vi "Round Settings.vi"(7 "DG_Number":i32, 8 "error in (no error)":errorcluster, 11 "Settings":T1={"Channel A"={"Delay (µs)"=0.013000000000000001, "Pulse Width (µs)"=0.019, "Output Modulo"=300, "Output Offset"=0, "Go Signal"=16, "Polarity"=TRUE, "Terminate"=FALSE}, "Channel B"={"Delay (µs)"=0.032, "Pulse Width (µs)"=0.019, "Output Modulo"=300, "Output Offset"=0, "Go Signal"=16, "Polarity"=TRUE, "Terminate"=FALSE}, "Channel C"={"Delay (µs)"=0.0, "Pulse Width (µs)"=0.01, "Output Modulo"=300, "Output Offset"=0, "Go Signal"=16, "Polarity"=TRUE, "Terminate"=FALSE}, "Channel D"={"Delay (µs)"=0.01, "Pulse Width (µs)"=0.01, "Output Modulo"=300, "Output Offset"=0, "Go Signal"=16, "Polarity"=TRUE, "Terminate"=FALSE}, "Channel E"={"Delay (µs)"=0.039999999999999994, "Pulse Width (µs)"=0.01, "Output Modulo"=300, "Output Offset"=1, "Go Signal"=16, "Polarity"=TRUE, "Terminate"=FALSE, "Disconnect"=FALSE, "Onto MsBus"=FALSE, "Input Positive"=TRUE}, "Channel F"={"Delay (µs)"=0.04999999999999999, "Pulse Width (µs)"=0.01, "Output Modulo"=300, "Output Offset"=1, "Go Signal"=16, "Polarity"=TRUE, "Terminate"=FALSE, "Disconnect"=FALSE, "Onto MsBus"=FALSE, "Input Positive"=TRUE}, "Clock Enable"=TRUE, "Ocillator Divider"=2, "Trigger Divider"=1, "Trigger Multiplier"=4, "Clock Source"=3, "Trigger Terminate"=TRUE, "Gate Terminate"=TRUE, "Trigger Level"=0.2, "Gate Level"=0.0, "Gate Delay (µs)"=-1.0, "MS Bus"=1, "Internal Clock (µs)"=0.0083333, "Stop Trigger"=1, "Gate Divider"=0, "Force Trigger (µs)"=-1.0, "Step Back Time (µs)"=-1.0, "Burst Counter"=1, "Positive Gate"=TRUE, "Trigger Source"=TRUE, "Gate Type"=TRUE, "Synchronize Gate"=FALSE, "Trigger Slope"=TRUE, "Stop on Preset"=FALSE, "Reset When Done"=TRUE, "Trigger Enable"=TRUE, "Gate AB"=0, "Gate CD"=0, "Gate EF"=0} {"Gate EF" items=["Normal"=0, "EF_OR"=1048576, "EF_AND"=2097152, "EF_XOR"=3145728]; "Gate CD" items=["Normal"=0, "CD_OR"=262144, "CD_AND"=524288, "CD_XOR"=786432]; "Gate AB" items=["Normal"=0, "AB_OR"=65536, "AB_AND"=131072, "AB_XOR"=196608]; "Step Back Time (µs)" min=-1.0 format="%.6f"; "Force Trigger (µs)" min=-1.0 format="%.6f"; "Gate Delay (µs)" min=-1.0 format="%.6f"; "Internal Clock (µs)" min=0.0 format="%.6f"; "MS Bus" format="%04x" items=["Local Primary"=1, "Local Secondary"=2, "Local Force"=4, "Resynchronize"=8, "Master Primary"=16, "Master Secondary"=32, "Master Force"=64, "System Clock"=128, "Delay Clock"=256, "Inhibit Local"=512, "Start Local"=1024, "Start Bus"=2048, "Step Back Local"=4096, "Step Back Bus"=8192, "Enable From E"=65536, "Enable From F"=131072, "Enable From Bus"=262144]; "Gate Level" min=-2.5 max=2.5 format="%.3g"; "Trigger Level" min=-2.5 max=2.5 format="%.3f"; "Clock Source" items=["Internal Oscillator"=1, "External Trigger"=2, "Trigger & Oscillator"=3, "Master Slave Bus"=4]; "Trigger Multiplier" min=1; "Trigger Divider" min=1; "Ocillator Divider" min=1; "Channel F"."Go Signal" format="%04x" items=["Loc Prim"=1, "Loc Sec"=2, "Loc Force"=4, "Resynch"=8, "Mas Prim"=16, "Mas Sec"=32, "Mas Force"=64, "Sys Clock"=128, "Delay Clock"=256, "Inhibit Local"=512, "Start Local"=1024, "Start Bus"=2048, "Step Back Loc"=4096, "Step Back Bus"=8192, "From E"=65536, "From F"=131072, "From Bus"=262144]; "Channel F"."Pulse Width (µs)" min=0.0 max=8947840.0 format="%.6f"; "Channel F"."Delay (µs)" min=0.0 format="%.6f"; "Channel E"."Go Signal" format="%04x" items=["Loc Prim"=1, "Loc Sec"=2, "Loc Force"=4, "Resynch"=8, "Mas Prim"=16, "Mas Sec"=32, "Mas Force"=64, "Sys Clock"=128, "Delay Clock"=256, "Inhibit Local"=512, "Start Local"=1024, "Start Bus"=2048, "Step Back Loc"=4096, "Step Back Bus"=8192, "From E"=65536, "From F"=131072, "From Bus"=262144]; "Channel E"."Pulse Width (µs)" min=0.0 max=8947840.0 format="%.6f"; "Channel E"."Delay (µs)" min=0.0 format="%.6f"; "Channel D"."Go Signal" format="%04x" items=["Loc Prim"=1, "Loc Sec"=2, "Loc Force"=4, "Resynch"=8, "Mas Prim"=16, "Mas Sec"=32, "Mas Force"=64, "Sys Clock"=128, "Delay Clock"=256, "Inhibit Local"=512, "Start Local"=1024, "Start Bus"=2048, "Step Back Loc"=4096, "Step Back Bus"=8192, "From E"=65536, "From F"=131072, "From Bus"=262144]; "Channel D"."Pulse Width (µs)" min=0.0 max=8947840.0 format="%.6f"; "Channel D"."Delay (µs)" min=0.0 format="%.6f"; "Channel C"."Go Signal" format="%04x" items=["Loc Prim"=1, "Loc Sec"=2, "Loc Force"=4, "Resynch"=8, "Mas Prim"=16, "Mas Sec"=32, "Mas Force"=64, "Sys Clock"=128, "Delay Clock"=256, "Inhibit Local"=512, "Start Local"=1024, "Start Bus"=2048, "Step Back Loc"=4096, "Step Back Bus"=8192, "From E"=65536, "From F"=131072, "From Bus"=262144]; "Channel C"."Pulse Width (µs)" min=0.0 max=8947840.0 format="%.6f"; "Channel C"."Delay (µs)" min=0.0 format="%.6f"; "Channel B"."Go Signal" format="%04x" items=["Loc Prim"=1, "Loc Sec"=2, "Loc Force"=4, "Resynch"=8, "Mas Prim"=16, "Mas Sec"=32, "Mas Force"=64, "Sys Clock"=128, "Delay Clock"=256, "Inhibit Local"=512, "Start Local"=1024, "Start Bus"=2048, "Step Back Loc"=4096, "Step Back Bus"=8192, "From E"=65536, "From F"=131072, "From Bus"=262144]; "Channel B"."Pulse Width (µs)" min=0.0 max=8947840.0 format="%.6f"; "Channel B"."Delay (µs)" min=0.0 format="%.6f"; "Channel A"."Go Signal" format="%04x" items=["Loc Prim"=1, "Loc Sec"=2, "Loc Force"=4, "Resynch"=8, "Mas Prim"=16, "Mas Sec"=32, "Mas Force"=64, "Sys Clock"=128, "Delay Clock"=256, "Inhibit Local"=512, "Start Local"=1024, "Start Bus"=2048, "Step Back Loc"=4096, "Step Back Bus"=8192, "From E"=65536, "From F"=131072, "From Bus"=262144]; "Channel A"."Pulse Width (µs)" min=0.0 max=8947840.0 format="%.6f"; "Channel A"."Delay (µs)" min=0.0 format="%.6f"}) -> (0 "error out":errorcluster, 3 "Settings":T1={"Channel A"={"Delay (µs)"=0.013000000000000001, "Pulse Width (µs)"=0.019, "Output Modulo"=300, "Output Offset"=0, "Go Signal"=16, "Polarity"=TRUE, "Terminate"=FALSE}, "Channel B"={"Delay (µs)"=0.032, "Pulse Width (µs)"=0.019, "Output Modulo"=300, "Output Offset"=0, "Go Signal"=16, "Polarity"=TRUE, "Terminate"=FALSE}, "Channel C"={"Delay (µs)"=0.0, "Pulse Width (µs)"=0.01, "Output Modulo"=300, "Output Offset"=0, "Go Signal"=16, "Polarity"=TRUE, "Terminate"=FALSE}, "Channel D"={"Delay (µs)"=0.01, "Pulse Width (µs)"=0.01, "Output Modulo"=300, "Output Offset"=0, "Go Signal"=16, "Polarity"=TRUE, "Terminate"=FALSE}, "Channel E"={"Delay (µs)"=0.039999999999999994, "Pulse Width (µs)"=0.01, "Output Modulo"=300, "Output Offset"=1, "Go Signal"=16, "Polarity"=TRUE, "Terminate"=FALSE, "Disconnect"=FALSE, "Onto MsBus"=FALSE, "Input Positive"=TRUE}, "Channel F"={"Delay (µs)"=0.04999999999999999, "Pulse Width (µs)"=0.01, "Output Modulo"=300, "Output Offset"=1, "Go Signal"=16, "Polarity"=TRUE, "Terminate"=FALSE, "Disconnect"=FALSE, "Onto MsBus"=FALSE, "Input Positive"=TRUE}, "Clock Enable"=TRUE, "Ocillator Divider"=2, "Trigger Divider"=1, "Trigger Multiplier"=4, "Clock Source"=3, "Trigger Terminate"=TRUE, "Gate Terminate"=TRUE, "Trigger Level"=0.2, "Gate Level"=0.0, "Gate Delay (µs)"=-1.0, "MS Bus"=1, "Internal Clock (µs)"=0.0083333, "Stop Trigger"=1, "Gate Divider"=0, "Force Trigger (µs)"=-1.0, "Step Back Time (µs)"=-1.0, "Burst Counter"=1, "Positive Gate"=TRUE, "Trigger Source"=TRUE, "Gate Type"=TRUE, "Synchronize Gate"=FALSE, "Trigger Slope"=TRUE, "Stop on Preset"=FALSE, "Reset When Done"=TRUE, "Trigger Enable"=TRUE, "Gate AB"=0, "Gate CD"=0, "Gate EF"=0} {"Gate EF" items=["Normal"=0, "EF_OR"=1048576, "EF_AND"=2097152, "EF_XOR"=3145728]; "Gate CD" items=["Normal"=0, "CD_OR"=262144, "CD_AND"=524288, "CD_XOR"=786432]; "Gate AB" items=["Normal"=0, "AB_OR"=65536, "AB_AND"=131072, "AB_XOR"=196608]; "Step Back Time (µs)" min=-1.0 format="%.6f"; "Force Trigger (µs)" min=-1.0 format="%.6f"; "Gate Delay (µs)" min=-1.0 format="%.6f"; "Internal Clock (µs)" min=0.0 format="%.6f"; "MS Bus" format="%04x" items=["Local Primary"=1, "Local Secondary"=2, "Local Force"=4, "Resynchronize"=8, "Master Primary"=16, "Master Secondary"=32, "Master Force"=64, "System Clock"=128, "Delay Clock"=256, "Inhibit Local"=512, "Start Local"=1024, "Start Bus"=2048, "Step Back Local"=4096, "Step Back Bus"=8192, "Enable From E"=65536, "Enable From F"=131072, "Enable From Bus"=262144]; "Gate Level" min=-2.5 max=2.5 format="%.3g"; "Trigger Level" min=-2.5 max=2.5 format="%.3f"; "Clock Source" items=["Internal Oscillator"=1, "External Trigger"=2, "Trigger & Oscillator"=3, "Master Slave Bus"=4]; "Trigger Multiplier" min=1; "Trigger Divider" min=1; "Ocillator Divider" min=1; "Channel F"."Go Signal" format="%04x" items=["Loc Prim"=1, "Loc Sec"=2, "Loc Force"=4, "Resynch"=8, "Mas Prim"=16, "Mas Sec"=32, "Mas Force"=64, "Sys Clock"=128, "Delay Clock"=256, "Inhibit Local"=512, "Start Local"=1024, "Start Bus"=2048, "Step Back Loc"=4096, "Step Back Bus"=8192, "From E"=65536, "From F"=131072, "From Bus"=262144]; "Channel F"."Pulse Width (µs)" min=0.0 max=8947840.0 format="%.6f"; "Channel F"."Delay (µs)" min=0.0 format="%.6f"; "Channel E"."Go Signal" format="%04x" items=["Loc Prim"=1, "Loc Sec"=2, "Loc Force"=4, "Resynch"=8, "Mas Prim"=16, "Mas Sec"=32, "Mas Force"=64, "Sys Clock"=128, "Delay Clock"=256, "Inhibit Local"=512, "Start Local"=1024, "Start Bus"=2048, "Step Back Loc"=4096, "Step Back Bus"=8192, "From E"=65536, "From F"=131072, "From Bus"=262144]; "Channel E"."Pulse Width (µs)" min=0.0 max=8947840.0 format="%.6f"; "Channel E"."Delay (µs)" min=0.0 format="%.6f"; "Channel D"."Go Signal" format="%04x" items=["Loc Prim"=1, "Loc Sec"=2, "Loc Force"=4, "Resynch"=8, "Mas Prim"=16, "Mas Sec"=32, "Mas Force"=64, "Sys Clock"=128, "Delay Clock"=256, "Inhibit Local"=512, "Start Local"=1024, "Start Bus"=2048, "Step Back Loc"=4096, "Step Back Bus"=8192, "From E"=65536, "From F"=131072, "From Bus"=262144]; "Channel D"."Pulse Width (µs)" min=0.0 max=8947840.0 format="%.6f"; "Channel D"."Delay (µs)" min=0.0 format="%.6f"; "Channel C"."Go Signal" format="%04x" items=["Loc Prim"=1, "Loc Sec"=2, "Loc Force"=4, "Resynch"=8, "Mas Prim"=16, "Mas Sec"=32, "Mas Force"=64, "Sys Clock"=128, "Delay Clock"=256, "Inhibit Local"=512, "Start Local"=1024, "Start Bus"=2048, "Step Back Loc"=4096, "Step Back Bus"=8192, "From E"=65536, "From F"=131072, "From Bus"=262144]; "Channel C"."Pulse Width (µs)" min=0.0 max=8947840.0 format="%.6f"; "Channel C"."Delay (µs)" min=0.0 format="%.6f"; "Channel B"."Go Signal" format="%04x" items=["Loc Prim"=1, "Loc Sec"=2, "Loc Force"=4, "Resynch"=8, "Mas Prim"=16, "Mas Sec"=32, "Mas Force"=64, "Sys Clock"=128, "Delay Clock"=256, "Inhibit Local"=512, "Start Local"=1024, "Start Bus"=2048, "Step Back Loc"=4096, "Step Back Bus"=8192, "From E"=65536, "From F"=131072, "From Bus"=262144]; "Channel B"."Pulse Width (µs)" min=0.0 max=8947840.0 format="%.6f"; "Channel B"."Delay (µs)" min=0.0 format="%.6f"; "Channel A"."Go Signal" format="%04x" items=["Loc Prim"=1, "Loc Sec"=2, "Loc Force"=4, "Resynch"=8, "Mas Prim"=16, "Mas Sec"=32, "Mas Force"=64, "Sys Clock"=128, "Delay Clock"=256, "Inhibit Local"=512, "Start Local"=1024, "Start Bus"=2048, "Step Back Loc"=4096, "Step Back Bus"=8192, "From E"=65536, "From F"=131072, "From Bus"=262144]; "Channel A"."Pulse Width (µs)" min=0.0 max=8947840.0 format="%.6f"; "Channel A"."Delay (µs)" min=0.0 format="%.6f"})   [LabVIEW 2009]
uses:
  Settings G08.ctl
panel:
  # "NOTICE -- YOU MUST LEAVE THIS NOTICE IN PLACE.  PER THE TERMS OF THE LICENSE BELOW, YOU MAY SUBLICENSE THIS SOFTWARE \nIN ANY WAY THAT DOES NOT CONFLICT WITH THIS LICENSE.\n\n### BSD License (http://www.opensource.org/licenses/bsd-license.php) Begin ###\n \nCopyright (c) 2011, Applied Energetics, http://www.appliedenergetics.com,\n                               Richard Schwerdtfeger, <rschwerdtfeger@appliedenergetics.com>\n\nAll rights reserved.\n\nRedistribution and use in source and binary forms, with or without modification, are permitted provided that the \nfollowing conditions are met:\n\n    * Redistributions of source code must retain the above copyright notice, this list of conditions and the following disclaimer.\n    * Redistributions in binary form must reproduce the above copyright notice, this list of conditions and the following disclaimer \n       in the documentation and/or other materials provided with the distribution.\n    * Neither the name of Richard Schwerdtfeger, Applied Energetics, Inc., nor the names of its contributors may be used to \n       endorse or promote products derived from this software without specific prior written permission.\n\nTHIS SOFTWARE IS PROVIDED BY THE COPYRIGHT HOLDERS AND CONTRIBUTORS \"AS IS\" AND ANY EXPRESS OR IMPLIED WARRANTIES, \nINCLUDING, BUT NOT LIMITED TO, THE IMPLIED WARRANTIES OF MERCHANTABILITY AND FITNESS FOR A PARTICULAR PURPOSE ARE \nDISCLAIMED. IN NO EVENT SHALL THE COPYRIGHT OWNER OR CONTRIBUTORS BE LIABLE FOR ANY DIRECT, INDIRECT, INCIDENTAL,\n SPECIAL, EXEMPLARY, OR CONSEQUENTIAL DAMAGES (INCLUDING, BUT NOT LIMITED TO, PROCUREMENT OF SUBSTITUTE GOODS OR \nSERVICES; LOSS OF USE, DATA, OR PROFITS; OR BUSINESS INTERRUPTION) HOWEVER CAUSED AND ON ANY THEORY OF LIABILITY, \nWHETHER IN CONTRACT, STRICT LIABILITY, OR TORT (INCLUDING NEGLIGENCE OR OTHERWISE) ARISING IN ANY WAY OUT OF THE USE \nOF THIS SOFTWARE, EVEN IF ADVISED OF THE POSSIBILITY OF SUCH DAMAGE.\n\n### BSD License End ###"
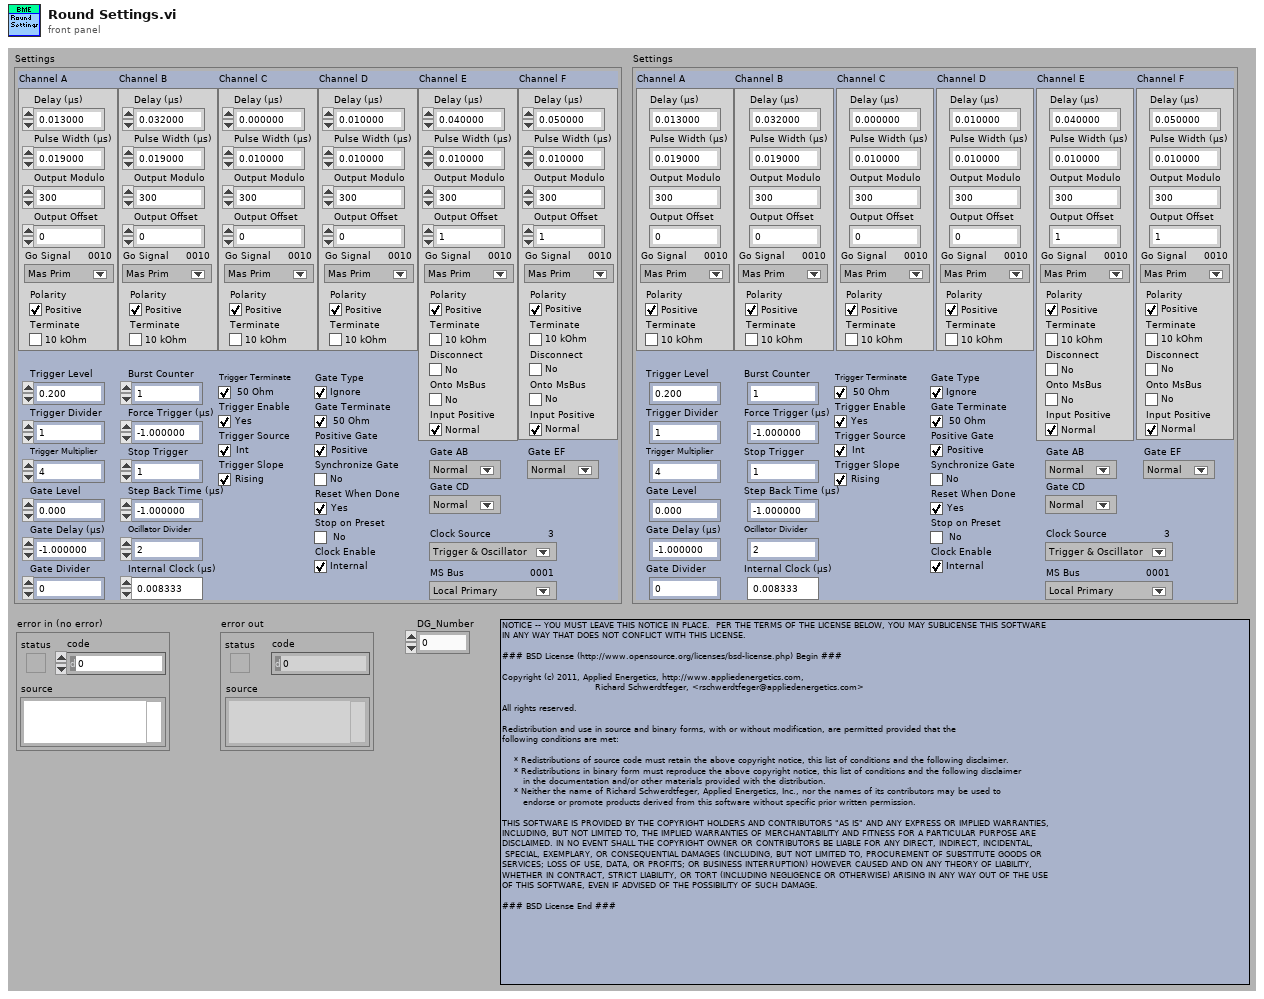
[diagram p1: front panel]
types:
  T1 = typedef "Settings G08.ctl" = cluster{"Channel A":cluster{"Delay (µs)":dbl, "Pulse Width (µs)":dbl, "Output Modulo":u32, "Output Offset":u32, "Go Signal":u32, "Polarity":bool, "Terminate":bool}, "Channel B":cluster{"Delay (µs)":dbl, "Pulse Width (µs)":dbl, "Output Modulo":u32, "Output Offset":u32, "Go Signal":u32, "Polarity":bool, "Terminate":bool}, "Channel C":cluster{"Delay (µs)":dbl, "Pulse Width (µs)":dbl, "Output Modulo":u32, "Output Offset":u32, "Go Signal":u32, "Polarity":bool, "Terminate":bool}, "Channel D":cluster{"Delay (µs)":dbl, "Pulse Width (µs)":dbl, "Output Modulo":u32, "Output Offset":u32, "Go Signal":u32, "Polarity":bool, "Terminate":bool}, "Channel E":cluster{"Delay (µs)":dbl, "Pulse Width (µs)":dbl, "Output Modulo":u32, "Output Offset":u32, "Go Signal":u32, "Polarity":bool, "Terminate":bool, "Disconnect":bool, "Onto MsBus":bool, "Input Positive":bool}, "Channel F":cluster{"Delay (µs)":dbl, "Pulse Width (µs)":dbl, "Output Modulo":u32, "Output Offset":u32, "Go Signal":u32, "Polarity":bool, "Terminate":bool, "Disconnect":bool, "Onto MsBus":bool, "Input Positive":bool}, "Clock Enable":bool, "Ocillator Divider":u32, "Trigger Divider":u32, "Trigger Multiplier":u32, "Clock Source":u32, "Trigger Terminate":bool, "Gate Terminate":bool, "Trigger Level":dbl, "Gate Level":dbl, "Gate Delay (µs)":dbl, "MS Bus":u32, "Internal Clock (µs)":dbl, "Stop Trigger":u32, "Gate Divider":u32, "Force Trigger (µs)":dbl, "Step Back Time (µs)":dbl, "Burst Counter":u32, "Positive Gate":bool, "Trigger Source":bool, "Gate Type":bool, "Synchronize Gate":bool, "Trigger Slope":bool, "Stop on Preset":bool, "Reset When Done":bool, "Trigger Enable":bool, "Gate AB":u32, "Gate CD":u32, "Gate EF":u32}
  T2 = cluster{"Delay (µs)":dbl, "Pulse Width (µs)":dbl, "Output Modulo":u32, "Output Offset":u32, "Go Signal":u32, "Polarity":bool, "Terminate":bool}
  T3 = cluster{"Delay (µs)":dbl, "Pulse Width (µs)":dbl, "Output Modulo":u32, "Output Offset":u32, "Go Signal":u32, "Polarity":bool, "Terminate":bool, "Disconnect":bool, "Onto MsBus":bool, "Input Positive":bool}
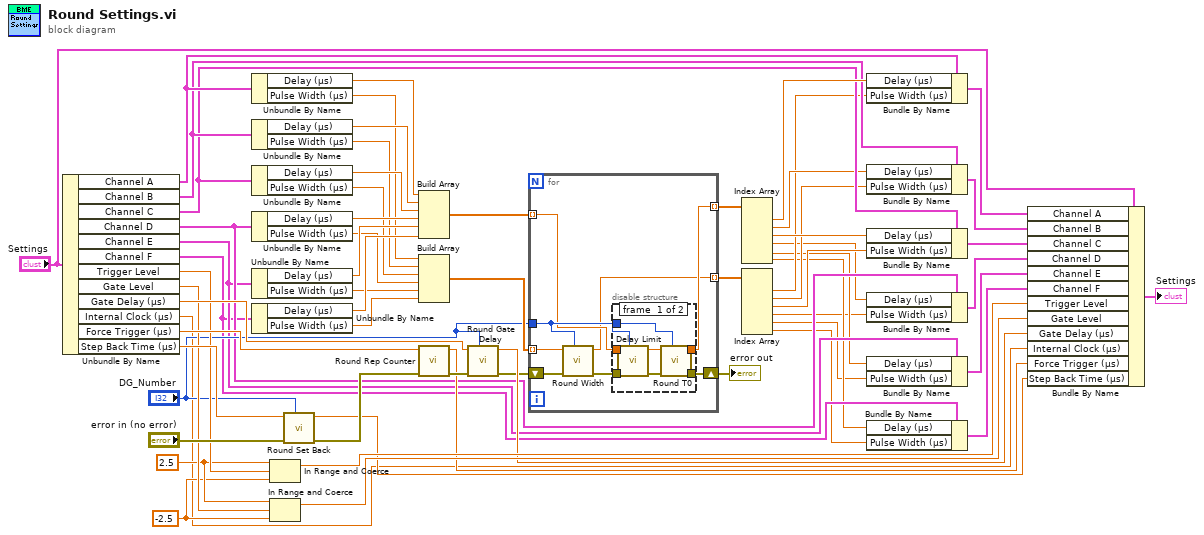
[diagram p0: block diagram]
diagram:
  w52 = -2.5 ("lower limit")
  w53 = 2.5 ("upper limit")
  n1 = Unbundle By Name("Settings") -> ("Channel A"=w25:T2, "Channel B"=w23:T2, "Channel C"=w22:T2, "Channel D"=w16:T2, "Channel E"=w15:T3, "Channel F"=w14:T3, "Trigger Level"=w55:dbl, "Gate Level"=w54:dbl, "Gate Delay (µs)"=w59:dbl, "Internal Clock (µs)"=w7:dbl, "Force Trigger (µs)"=w56:dbl, "Step Back Time (µs)"=w60:dbl)
  n2 = Unbundle By Name(w25) -> ("Delay (µs)"=w44:dbl, "Pulse Width (µs)"=w38:dbl)
  n3 = Unbundle By Name(w23) -> ("Delay (µs)"=w43:dbl, "Pulse Width (µs)"=w37:dbl)
  n4 = Unbundle By Name(w22) -> ("Delay (µs)"=w42:dbl, "Pulse Width (µs)"=w36:dbl)
  n5 = Unbundle By Name(w16) -> ("Delay (µs)"=w41:dbl, "Pulse Width (µs)"=w35:dbl)
  n6 = Unbundle By Name(w15) -> ("Delay (µs)"=w40:dbl, "Pulse Width (µs)"=w34:dbl)
  n7 = Unbundle By Name(w14) -> ("Delay (µs)"=w39:dbl, "Pulse Width (µs)"=w33:dbl)
  n8 = In Range and Coerce(upper limit=w53, x=w55, lower limit=w52) -> (coerced(x)=w49:dbl)  [unwired: 1 out]
  n9 = In Range and Coerce(upper limit=w53, x=w54, lower limit=w52) -> (coerced(x)=w48:dbl)  [unwired: 1 out]
  n10 = call "Round Set Back.vi"("DG_Number"="DG_Number", "error in (no error)"="error in (no error)", "Step Back Time (µs)"=w60) -> ("error out"=w58:errorcluster, "Step Back Time (µs)"=w45:dbl)  [unwired: 2 in, 5 out]
  n11 = Build Array(w44, w43, w42, w41, w40, w39) -> (w30:dbl[])
  n12 = Build Array(w38, w37, w36, w35, w34, w33) -> (w31:dbl[])
  n13 = call "Round Rep Counter.vi"("error in (no error)"=w58, "In Value"=w56) -> ("error out"=w57:errorcluster, "Result"=w46:dbl)  [unwired: 1 in, 7 out]
  n14 = call "Round Gate Delay.vi"("DG_Number"="DG_Number", "error in (no error)"=w57, "Gate Delay (µs)"=w59) -> ("error out"=w32:errorcluster, "Gate Delay (µs)"=w47:dbl)  [unwired: 2 in, 5 out]
  n15 = for {
    shift-right: [w67] -> w29
    shift-left: w32 -> [w69]
    tunnel: w31 -> [w65] mode=indexing
    tunnel: w30 -> [w64] mode=indexing
    tunnel: "DG_Number" -> [w66]
    tunnel: [w63] -> w27 mode=indexing
    tunnel: [w62] -> w26 mode=indexing
    n16 = call "Round Width.vi"("DG_Number"=w66, "error in (no error)"=w69, "Pulse Width (µs)"=w65) -> ("error out"=w68:errorcluster, "Pulse Width (µs)"=w62:dbl)  [unwired: 7 out]
    n17 = disable-structure shown="Enabled" {
      disable-tunnel: w68 -> [w76 w78]
      disable-tunnel: [w74 w78] -> w67
      disable-tunnel: w66 -> [w73 _]
      disable-tunnel: w64 -> [w72 w77]
      disable-tunnel: [w70 w77] -> w63
      frame #0 {
        n18 = call "Delay Limit.vi"("DG Number"=w73, "error in (no error)"=w76, "In Value"=w72) -> ("error out"=w75:errorcluster, "Delay Limit"=w71:dbl)  [unwired: 7 in]
        n19 = call "Round T0.vi"("DG Number"=w73, "error in (no error)"=w75, "In Value"=w71) -> ("error out"=w74:errorcluster, "Result"=w70:dbl)  [unwired: 7 in]
      }
      frame #1 {
      }
    }
  }
  "error out" <- w29
  n20 = Index Array(array=w27) -> (element #1=w24:dbl, element #2=w21:dbl, element #3=w20:dbl, element #4=w6:dbl, element #5=w5:dbl, element #6=w4:dbl)  [unwired: 6 in]
  n21 = Index Array(array=w26) -> (element #1=w19:dbl, element #2=w18:dbl, element #3=w17:dbl, element #4=w3:dbl, element #5=w2:dbl, element #6=w1:dbl)  [unwired: 6 in]
  n22 = Bundle By Name(cluster=w25, "Delay (µs)"=w24, "Pulse Width (µs)"=w19) -> (w13:T2)
  n23 = Bundle By Name(cluster=w23, "Delay (µs)"=w21, "Pulse Width (µs)"=w18) -> (w12:T2)
  n24 = Bundle By Name(cluster=w22, "Delay (µs)"=w20, "Pulse Width (µs)"=w17) -> (w11:T2)
  n25 = Bundle By Name(cluster=w16, "Delay (µs)"=w6, "Pulse Width (µs)"=w3) -> (w10:T2)
  n26 = Bundle By Name(cluster=w15, "Delay (µs)"=w5, "Pulse Width (µs)"=w2) -> (w9:T3)
  n27 = Bundle By Name(cluster=w14, "Delay (µs)"=w4, "Pulse Width (µs)"=w1) -> (w8:T3)
  n28 = Bundle By Name(cluster="Settings", "Channel A"=w13, "Channel B"=w12, "Channel C"=w11, "Channel D"=w10, "Channel E"=w9, "Channel F"=w8, "Trigger Level"=w49, "Gate Level"=w48, "Gate Delay (µs)"=w47, "Internal Clock (µs)"=w7, "Force Trigger (µs)"=w46, "Step Back Time (µs)"=w45) -> (→"Settings":T1)
